vi "Set Tree custom symbols.vi"(11 "TreeControl in":refnum<vi>) -> (3 "TreeControl out":refnum<vi>)   [LabVIEW 2019, in "Panther Dashboard.lvlib"]
uses:
  Panther Dashboard.lvlib
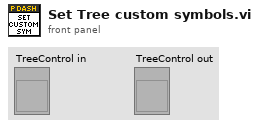
[diagram p1: front panel]
types:
  T1 = typedef "imagedata.ctl" = cluster{"image type":i32, "image depth":i32, "image":u8[], "mask":u8[], "colors":u32[], "Rectangle":cluster{"left":i16, "top":i16, "right":i16, "bottom":i16}}
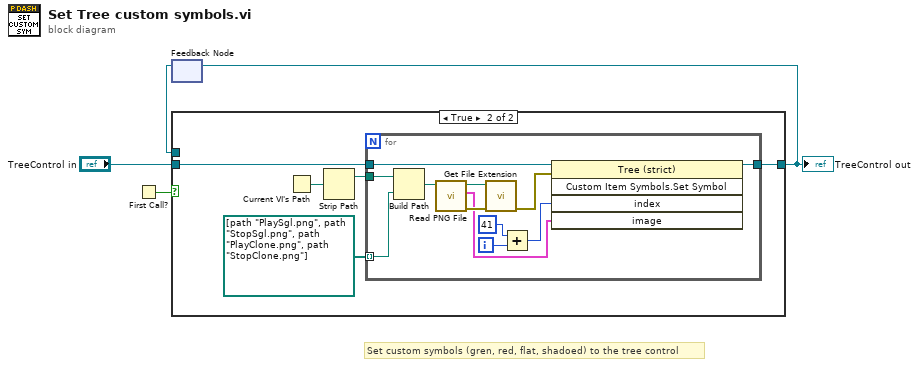
[diagram p0: block diagram]
diagram:
  # "Set custom symbols (gren, red, flat, shadoed) to the tree control"
  n1 = First Call?() -> (First Call?: T/F=w1:bool)
  n2 = feedback #1() -> (w4:refnum<vi>)  [unwired: 1 in]
  n3 = case shown="True" w1 {
    tunnel: [w5 w8] -> w3
    tunnel: "TreeControl in" -> [_ w6]
    tunnel: w4 -> [w5 _]
    frame False {
    }
    frame True {
      n4 = Current VI's Path() -> (path=w10:path)
      n5 = Strip Path(path=w10) -> (stripped path=w7:path)  [unwired: 1 out]
      n6 = for {
        tunnel: w7 -> [w19]
        tunnel: path[] [path "PlaySgl.png", path "StopSgl.png", path "PlayClone.png", path "StopClone.png"] ("name or relative path") -> [w18] mode=indexing
        tunnel: w6 -> [w12]
        tunnel: [w11] -> w8
        i -> [w15]
        n7 = Build Path(base path=w19, name or relative path=w18) -> (appended path=w17:path)
        n8 = call <vilib>:"Read PNG File.vi"("path to PNG file"=w17) -> ("error out"=w22:errorcluster, "image data"=w14:T1, "path"=w20:path)  [unwired: 8 in]
        n9 = call <vilib>:"Get File Extension.vi"("error in (no error)"=w22, "file"=w20) -> ("error out"=w21:errorcluster)  [unwired: 5 in, 4 out]
        n10 = Add(x=41 ("Index"), y=w15) -> (x+y=w13:i32)
        n11 = invoke on="Invoke Node" class="Tree (strict)" method="Custom Item Symbols.Set Symbol"(reference=w12, error in=w21, "index"=w13, "image"=w14) -> (reference out=w11:refnum<vi>)  [unwired: 1 in, 4 out]
      }
    }
  }
  "TreeControl out" <- w3
  n12 = feedback-in #1(w3) -> ()
